vi "examen de programacion 2.vi"() -> ()   [LabVIEW 2017]
uses:
  <vilib>/Analysis/_algsub.llb/Real Vector Norm.vi
  <vilib>/Analysis/baseanly.llb/Real Determinant.vi
  <vilib>/Analysis/baseanly.llb/Real Dot Product.vi
  <vilib>/Analysis/NI_AALBase.lvlib
  <vilib>/Analysis/NI_AALPro.lvlib
panel:
  out "Grados":i32=360
  out "Angulos":dbl[](array[numeric])=[-112.50644475393963, -75.66218987221903, 49.837630838654576, -104.7425770136151, -116.92643803236844]
  out "VEC B":dbl[][](array[numeric])=[[1.6165274287918932, 0.6697999999999666], [-0.5471576390030517, 3.8117999999999626], [0.830724027196653, 0.9333999999999634], [-1.6646673382299744, 0.8454999999999586], [0.0, -2.7800000000000438]]
  out "VEC A":dbl[][](array[numeric])=[[-9.138037038169955e-07, -2.7800000000000438], [1.6165274287918932, 0.6697999999999666], [-0.5471576390030517, 3.8117999999999626], [0.830724027196653, 0.9333999999999634], [-1.6646673382299744, 0.8454999999999586]]
  in  "Longitude py":dbl=-65.75479999999996
  in  "Latitude px":dbl=5.35343
  out "No Pertenece":bool
  out "Pertenece":bool=TRUE
  in  "Longitude":dbl[](array[numeric])=[-68.5348, -65.085, -61.943, -64.8214, -64.9093, -68.5348]
  in  "Latitude":dbl[](array[numeric])=[5.3534290861962965, 6.9699574287918935, 4.806272360996949, 6.184154027196653, 3.688762661770026, 5.35343]
  out "XY Graph":cluster{"p1x":dbl[], "p1y":dbl[]}[](graph)=[{"p1x"=[5.3534290861962965, 6.9699574287918935, 4.806272360996949, 6.184154027196653, 3.688762661770026, 5.35343], "p1y"=[-68.5348, -65.085, -61.943, -64.8214, -64.9093, -68.5348]}, {"p1x"=[5.35343], "p1y"=[-65.75479999999996]}]
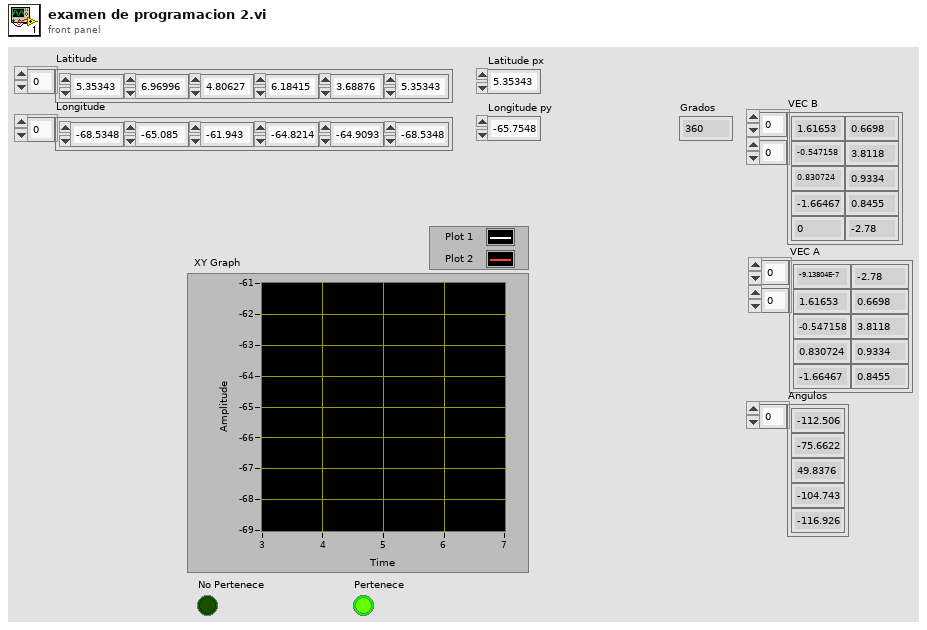
[diagram p1: front panel]
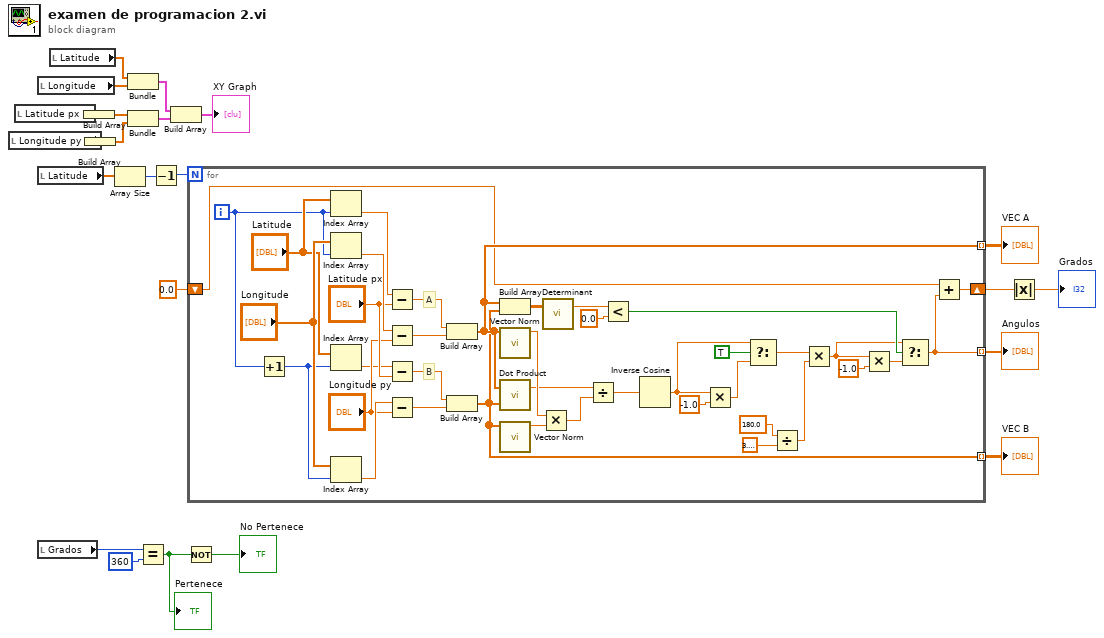
[diagram p0: block diagram]
diagram:
  n1 = local read "Longitude py"() -> (w15:dbl)
  n2 = local read "Latitude px"() -> (w17:dbl)
  n3 = local read "Longitude"() -> (w21:dbl[])
  n4 = local read "Latitude"() -> (w18:dbl[])
  n5 = local read "Grados"() -> (w6:i32)
  n6 = local read "Latitude"() -> (w22:dbl[])
  n7 = Build Array(w17) -> (w16:dbl[])
  n8 = Build Array(w15) -> (w14:dbl[])
  n9 = Array Size(array=w18) -> (size(s)=w8:i32)
  n10 = Bundle("Latitude"=w22, "Longitude"=w21) -> (w20:cluster{"Latitude":dbl[], "Longitude":dbl[]})  [unwired: 1 in]
  n11 = Bundle(w16, w14) -> (w13:cluster{dbl[], dbl[]})  [unwired: 1 in]
  n12 = Equal?(x=w6, y=360) -> (x = y?=w4:bool)
  "Pertenece" <- w4
  n13 = Decrement(x=w8) -> (x-1=w7:i32)
  n14 = Build Array(w20, w13) -> (→"XY Graph":cluster{"Latitude":dbl[], "Longitude":dbl[]}[])
  n15 = Not(x=w4) -> (.not. x?=→"No Pertenece":bool)
  n16 = for {
    N: w7 -> [_]
    shift-right: [w49] -> w2
    shift-left: 0.0 -> [w33]
    tunnel: [w37] -> w12 mode=indexing
    tunnel: [w36] -> w11 mode=indexing
    tunnel: [w28] -> w3 mode=indexing
    i -> [w51]
    # "B"
    # "A"
    n17 = Increment(x=w51) -> (x+1=w50:i32)
    n18 = Index Array(array="Latitude", index=w51) -> (element=w40:dbl)
    n19 = Index Array(array="Longitude", index=w51) -> (element=w61:dbl)
    n20 = Index Array(array="Latitude", index=w50) -> (element=w39:dbl)
    n21 = Index Array(array="Longitude", index=w50) -> (element=w58:dbl)
    n22 = Subtract(x=w40, y="Latitude px") -> (x-y=w44:dbl)
    n23 = Subtract(x=w61, y="Longitude py") -> (x-y=w55:dbl)
    n24 = Subtract(x=w39, y="Latitude px") -> (x-y=w45:dbl)
    n25 = Subtract(x=w58, y="Longitude py") -> (x-y=w54:dbl)
    n26 = Build Array(w44, w55) -> (w37:dbl[])
    n27 = Build Array(w45, w54) -> (w36:dbl[])
    n28 = Build Array(w37, w36) -> (w35:dbl[][])
    n29 = call-poly <vilib>:"Vector Norm.vi"("Input Vector"=w37) -> ("norm"=w53:dbl)  [unwired: 9 in, 1 out]
    n30 = call-poly <vilib>:"Dot Product.vi"("Y Vector"=w36, "X Vector"=w37) -> ("X * Y"=w27:dbl)  [unwired: 1 out]
    n31 = call-poly <vilib>:"Vector Norm.vi"("Input Vector"=w36) -> ("norm"=w52:dbl)  [unwired: 9 in, 1 out]
    n32 = Multiply(x=w53, y=w52) -> (x*y=w25:dbl)
    n33 = call-poly <vilib>:"Determinant.vi"("Input Matrix"=w35) -> ("determinant"=w24:dbl)  [unwired: 1 in, 1 out]
    n34 = Divide(x=w27, y=w25) -> (x/y=w26:dbl)
    n35 = Less?(x=w24, y=0.0) -> (x < y?=w34:bool)
    n36 = Inverse Cosine(1:w26) -> (0:w23:dbl)
    n37 = Multiply(x=w23, y=-1.0) -> (x*y=w43:dbl)
    n38 = Select(t=w23, s=TRUE, f=w43) -> (s? t:f=w41:dbl)
    n39 = Divide(x=180.0, y=3.141592653589793) -> (x/y=w48:dbl)
    n40 = Multiply(x=w41, y=w48) -> (x*y=w31:dbl)
    n41 = Multiply(x=w31, y=-1.0) -> (x*y=w29:dbl)
    n42 = Select(t=w31, s=w34, f=w29) -> (s? t:f=w28:dbl)
    n43 = Add(x=w33, y=w28) -> (x+y=w49:dbl)
  }
  "VEC A" <- w12
  "VEC B" <- w11
  "Angulos" <- w3
  n44 = Absolute Value(x=w2) -> (abs(x)=→"Grados":dbl)
